vi "UIMessageProgessPercent.vi"   [LabVIEW 2017]
uses:
  Support/MessageAPI/UIMessage.ctl
  SendMessage/SendMessage.lvclass
types:
  T1 = typedef "UIMessage.ctl" = cluster{"EventCode":i32, "Numeric":dbl, "String":string, "Variant":variant}
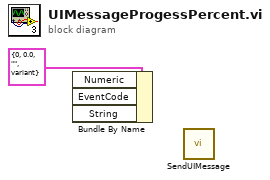
[diagram p0: block diagram]
diagram:
  n1 = Bundle By Name(cluster=T1 {"EventCode"=0, "Numeric"=0.0, "String"="", "Variant"=variant} ("UIMsg")) -> (w4:T1, "Numeric"=w1:dbl, "EventCode"=w2:i32, "String"=w3:string)
  n2 = call-dynamic "SendUIMessage.vi"() -> ()  [unwired: 10 in, 2 out]
